vi "Get Frame.vi"(8 "error in (no error)":errorcluster, 11 "Item Ref in":T1 format="%.0x") -> (0 "error out":errorcluster, 2 "PID In":T2 {"Signals"."Byte Order" items=["Little Endian", "Big Endian"]; "Signals"."Data Type" items=["Signed", "Unsigned", "IEEE Float"]}, 3 "Item Ref out":T1 format="%.0x")   [LabVIEW 2015, in "Diagnostics Addon System Explorer.lvlib"]
uses:
  System Explorer/Diagnostics Addon System Explorer.lvlib
  Frame Parameters.ctl
  Signal Parameters.ctl
  <vilib>/NI Veristand/Custom Device API/Custom Device Item Ref.ctl
  FG Action.ctl
  Signal Parameters FG.vi
  <vilib>/NI Veristand/Custom Device API/NI VeriStand - Get Custom Device Channel Data.vi
  <vilib>/NI Veristand/Custom Device API/NI VeriStand - Get Item Description.vi
  <vilib>/NI Veristand/Custom Device API/NI VeriStand - Get Item Property.vi
  <vilib>/NI Veristand/Custom Device API/Get Item Property (String).vi
  <vilib>/NI Veristand/Custom Device API/Get Item Property (Double).vi
  <vilib>/NI Veristand/Custom Device API/Get Item Property (U32).vi
  <vilib>/NI Veristand/Custom Device API/NI VeriStand - Set Item Property.vi
  <vilib>/NI Veristand/Custom Device API/Set Item Property (String).vi
  <vilib>/NI Veristand/Custom Device API/Set Item Property (Double).vi
  <vilib>/NI Veristand/Custom Device API/Set Item Property (U32).vi
  GUID Lookup.vi
  <vilib>/NI Veristand/Custom Device API/NI VeriStand - Get Item Children.vi
  <vilib>/NI Veristand/Custom Device API/Custom Device API.lvlib
  Diagnostics Addon Shared.lvlib
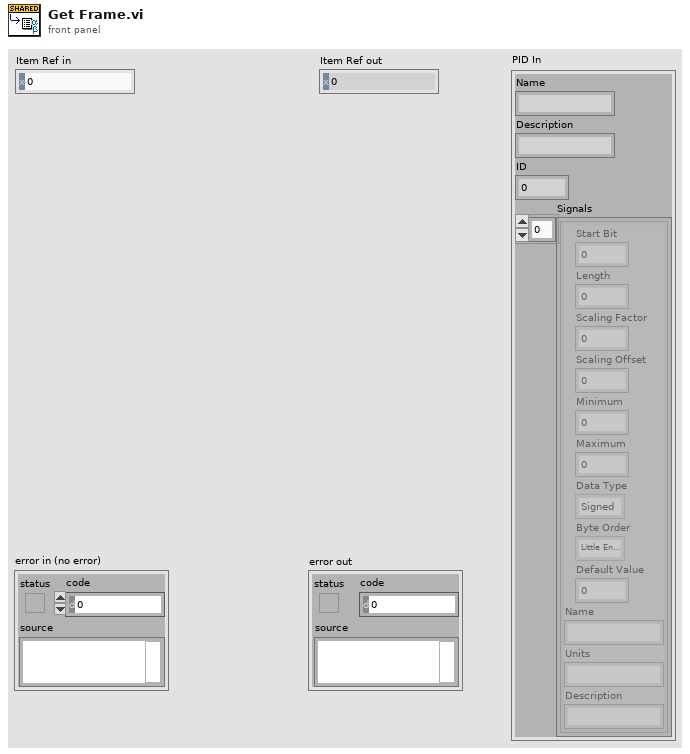
[diagram p1: front panel]
types:
  T1 = typedef "Custom Device API.lvlib/Custom Device Item Ref.ctl" = u64
  T2 = typedef "Diagnostics Addon Shared.lvlib/Frame Parameters.ctl" = cluster{"Name":string, "Description":string, "ID":u16, "Signals":T3[]}
  T3 = typedef "Diagnostics Addon Shared.lvlib/Signal Parameters.ctl" = cluster{"Start Bit":u8, "Length":u8, "Scaling Factor":dbl, "Scaling Offset":dbl, "Minimum":dbl, "Maximum":dbl, "Data Type":u32, "Byte Order":u32, "Default Value":dbl, "Name":string, "Units":string, "Description":string}
  T4 = typedef "Diagnostics Addon System Explorer.lvlib/FG Action.ctl" = enum16{"Get", "Set"}
  T5 = typedef "Custom Device API.lvlib/Custom Device Item Info.ctl" = cluster{"Name":string, "Is Channel":bool, "GUID":string, "Is Waveform":bool}
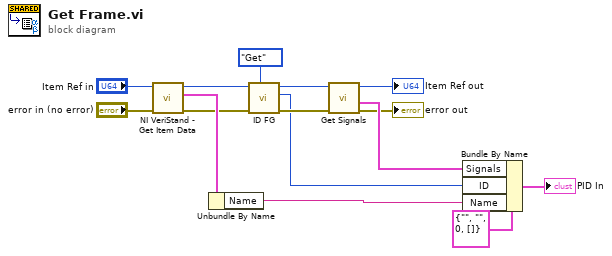
[diagram p0: block diagram]
diagram:
  n1 = call <vilib>:"NI VeriStand - Get Item Data.vi"("error in (no error)"="error in (no error)", "Item Ref in"="Item Ref in") -> ("error out"=w13:errorcluster, "Item Info"=w15:T5, "Item Ref out"=w14:T1)  [unwired: 7 out]
  n2 = Unbundle By Name(w15) -> ("Name"=w10:string)
  n3 = call "ID FG.vi"("Action"=FG_Action."Get", "error in (no error)"=w13, "Device Item Ref in"=w14) -> ("error out"=w12:errorcluster, "ID"=w8:u32, "Device Item Ref out"=w11:T1)  [unwired: 6 in]
  n4 = call "Get Signals.vi"("error in (no error)"=w12, "Device Item Ref out"=w11) -> ("error out"=→"error out":errorcluster, "Parameters"=w7:T3[], "Item Ref out"=→"Item Ref out":T1)  [unwired: 6 in, 1 out]
  n5 = Bundle By Name(cluster=T2 {"Name"="", "Description"="", "ID"=0, "Signals"=[]} ("PID In"), "Signals"=w7, "ID"=w8, "Name"=w10) -> (→"PID In":T2)
